vi "Basic_pn.vi"() -> ()   [LabVIEW 2019, in "GettingStarted_5775_Host.lvlib"]
uses:
  GettingStarted_5775_Host.lvlib
  <vilib>/userDefined/High Color/nirio_resource_hc.ctl
  <instrlib>/FlexRIO/API/Host/v1/NI FlexRIO/API/Reference Clock Source.ctl
  <instrlib>/FlexRIO/API/Host/v1/NI FlexRIO/API/Configure Reference Clock.vi
  <instrlib>/FlexRIO/API/Host/v1/NI FlexRIO/API/Get Property Reference - Fpga Small.vi
  <instrlib>/FlexRIO/API/Host/v1/NI FlexRIO/API/Configure Analog Start Trigger.vi
  <instrlib>/FlexRIO/API/Host/v1/NI FlexRIO/API/Configure Digital Edge Start Trigger.vi
  <instrlib>/FlexRIO/API/Host/v1/NI FlexRIO/API/Configure Immediate Start Trigger.vi
  <instrlib>/FlexRIO/API/Host/v1/NI FlexRIO/API/Read Stream 1D WDT.vi
  <vilib>/measure/maspectr.llb/FFT Power Spectrum and PSD for N Chan.vi
  <vilib>/FPGAPlugInAG/Dynamic/niLvFpga_Close_Dynamic.vi
  <vilib>/rvi/interface/nirviCloseFPGA/nirviCloseFPGA.xnode
  <instrlib>/FlexRIO/API/Host/v1/NI FlexRIO API v1.lvlib
  <resource>/objmgr/niflexrioapiStream.rc
  <vilib>/measure/NI_MAPro.lvlib
panel:
  in  "reference clock source":T1 items=["Default", "Onboard", "PXI_Clk10", "External", "None", "Baseboard Reference"]
  out "Sample Rate":dbl=3200000000.0 format="%#_6p"
  in  "ADC Interleaving Factor":i32=1 min=0 max=2 step=1
  in  "AI num samples":u64=320 step=16
  in  "AI channels":string="AI0,AI1"
  out "Device Power":dbl(slide) scale=-1.0..58.0 scale format="%#_3p"
  out "FPGA Temperature":dbl(slide) scale=0.0..100.0 scale format="%#_3p"
  in  "Trigger Type":enum32{"Immediate", "Analog", "Digital"}(tab)
  in  "trigger channel":string="AI0"
  in  "rising edge?":bool=TRUE
  in  "level (V)":dbl format="%#_3p"
  in  "hysteresis (V)":dbl format="%#_3p"
  in  "digital trigger source":string(combo)
  in  "stop":bool
  in  "Bitfile path":path
  in  "Waveform Tab Control":enum32{"AI Time Domain", "AI Frequency Domain"}(tab)
  out "Waveform Graph":waveform(dbl)[](graph)
  out "FFT":cluster{"f0":dbl, "df":dbl, "magnitude":dbl[]}[](graph) caption="Waveform Graph"
  out "error out":errorcluster
  out "Limit (W)":dbl
  out "Power (W)":dbl
  out "Limit (C)":dbl
  out "Temp (C)":dbl format="%#_4p"
  in  "RIO Device":T2
  # "Overview: Configure an acquisition for a FlexRIO target and transfer the data to the host using the FlexRIO Host API.  Loop an output waveform\nRequirements: FlexRIO\nInstructions: \n 1. Select the RIO Device that corresponds to the FlexRIO target. \n 2. Select the bitfile path that corresponds to your device\n 3. Optionally configure the clocking, stream, and trigger. \n 4. Run the VI"
  # "Resource Configuration"
  # "Clocking configuration"
  # "Input Waveform Configuration"
  # "Device Monitoring"
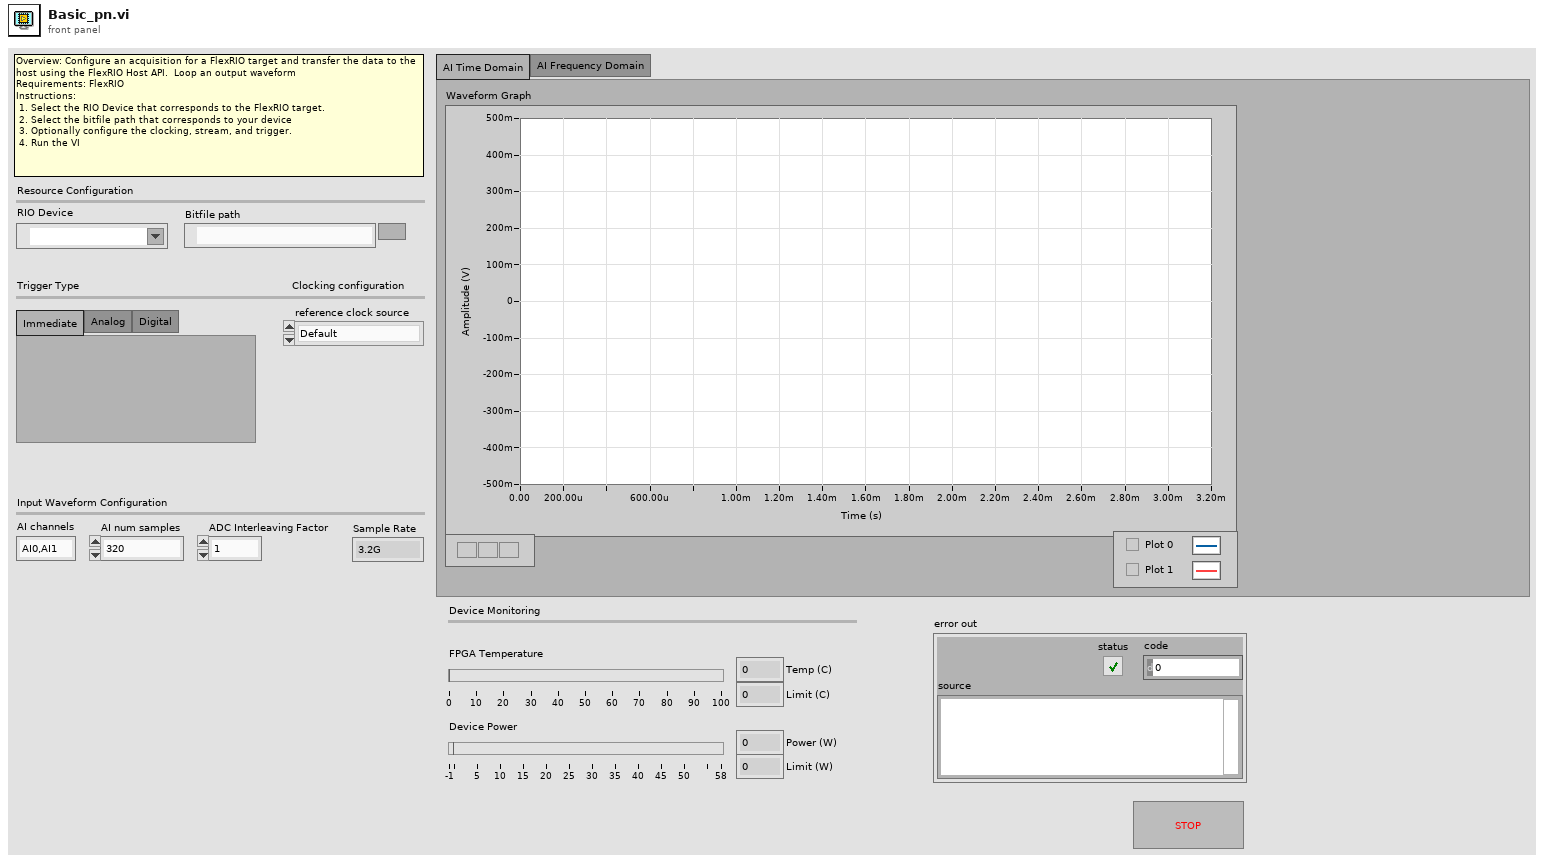
[diagram p1: front panel]
types:
  T1 = typedef "NI FlexRIO API v1.lvlib/Reference Clock Source.ctl" = i32
  T2 = typedef "nirio_resource_hc.ctl" = tag
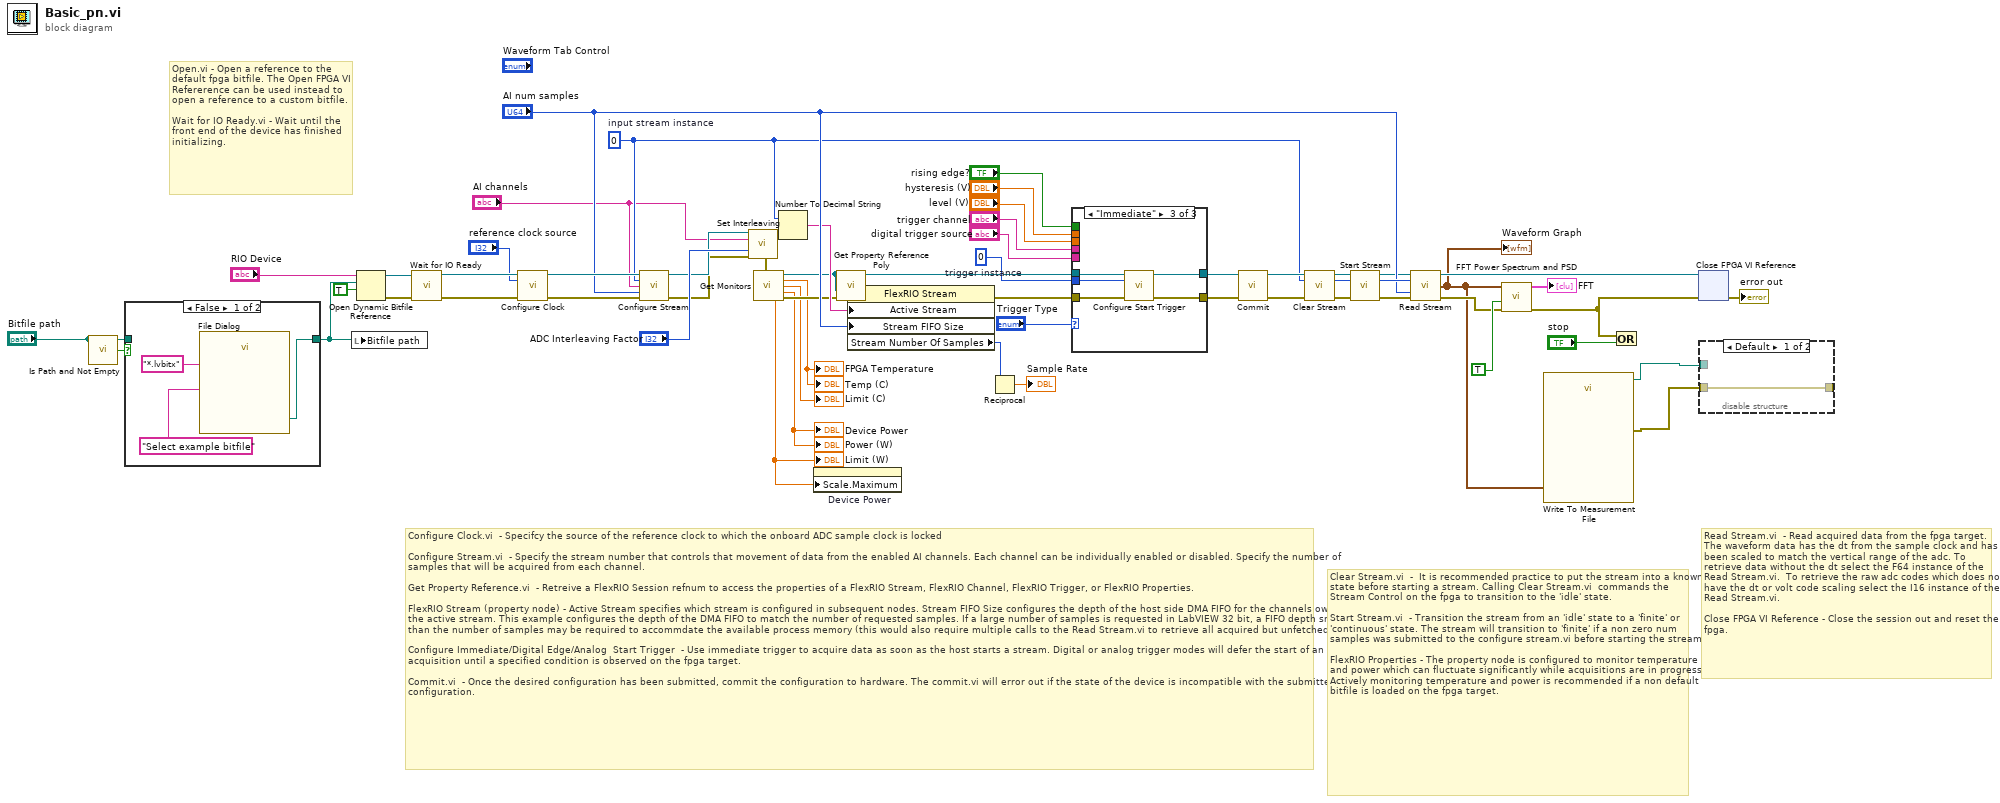
[diagram p0: block diagram]
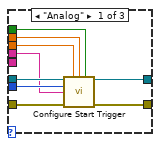
[diagram p2: hidden frame]
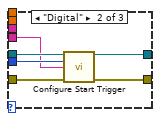
[diagram p3: hidden frame]
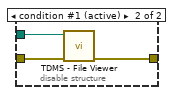
[diagram p4: hidden frame]
diagram:
  w32 = u32 0  # trigger instance
  w21 = u32 0  # input stream instance
  # "Read Stream.vi  - Read acquired data from the fpga target. The waveform data has the dt from the sample clock and has been scaled to match the vertical range of the adc. To retrieve data without the dt select the F64 instance of the Read Stream.vi.  To retrieve the raw adc codes which does not have the dt or volt code scaling select the I16 instance of the Read Stream.vi.  \n\nClose FPGA VI Reference - Close the session out and reset the fpga."
  # "Clear Stream.vi  -  It is recommended practice to put the stream into a known state before starting a stream. Calling Clear Stream.vi  commands the Stream Control on the fpga to transition to the 'idle' state.\n\nStart Stream.vi  - Transition the stream from an 'idle' state to a 'finite' or 'continuous' state. The stream will transition to 'finite' if a non zero num samples was submitted to the configure stream.vi before starting the stream.  \n\nFlexRIO Properties - The property node is configured to monitor temperature and power which can fluctuate significantly while acquisitions are in progress. Actively monitoring temperature and power is recommended if a non default bitfile is loaded on the fpga target."
  # "Configure Clock.vi  - Specifcy the source of the reference clock to which the onboard ADC sample clock is locked\n\nConfigure Stream.vi  - Specify the stream number that controls that movement of data from the enabled AI channels. Each channel can be individually enabled or disabled. Specify the number of samples that will be acquired from each channel. \n\nGet Property Reference.vi  - Retreive a FlexRIO Session refnum to access the properties of a FlexRIO Stream, FlexRIO Channel, FlexRIO Trigger, or FlexRIO Properties.\n\nFlexRIO Stream (property node) - Active Stream specifies which stream is configured in subsequent nodes. Stream FIFO Size configures the depth of the host side DMA FIFO for the channels owned by the active stream. This example configures the depth of the DMA FIFO to match the number of requested samples. If a large number of samples is requested in LabVIEW 32 bit, a FIFO depth smaller than the number of samples may be required to accommdate the available process memory (this would also require multiple calls to the Read Stream.vi to retrieve all acquired but unfetched data). \n\nConfigure Immediate/Digital Edge/Analog  Start Trigger  - Use immediate trigger to acquire data as soon as the host starts a stream. Digital or analog trigger modes will defer the start of an acquisition until a specified condition is observed on the fpga target. \n\nCommit.vi  - Once the desired configuration has been submitted, commit the configuration to hardware. The commit.vi will error out if the state of the device is incompatible with the submitted configuration."
  # "Open.vi - Open a reference to the default fpga bitfile. The Open FPGA VI Refererence can be used instead to open a reference to a custom bitfile.\n\nWait for IO Ready.vi - Wait until the front end of the device has finished initializing."
  n1 = call <vilib>:"Is Path and Not Empty.vi"("path"="Bitfile path") -> ("Is Path and Not Empty?"=w49:bool)  [unwired: 4 in]
  n2 = case shown="False" w49 {
    tunnel: "Bitfile path" -> [_ w63]
    tunnel: [w61 w63] -> w48
    frame False {
      n3 = call "File Dialog"("prompt"="Select example bitfile", "pattern (all files)"="*.lvbitx") -> ("selected path"=w61:path)  [unwired: 10 in, 3 out]
    }
    frame True {
    }
  }
  n4 = local write "Bitfile path"(w48) -> ()
  n5 = Open Dynamic Bitfile Reference(0:"RIO Device", 1:w48, 2:TRUE ("Run When Loaded")) -> (5:w55:refnum<k20>, 8:w56:errorcluster)  [unwired: 2 in]
  n6 = call <instrlib>:"Wait for IO Ready.vi"("fpga interface in"=w55, "error in"=w56) -> ("fpga interface out"=w57:refnum<k20>, "error out"=w58:errorcluster)  [unwired: 10 in, 2 out]
  n7 = call-poly <instrlib>:"Configure Clock.vi"("fpga interface in"=w57, "reference clock source"="reference clock source", "error in"=w58) -> ("fpga interface out"=w38:refnum<k20>, "error out"=w37:errorcluster)  [unwired: 11 in]
  n8 = call <instrlib>:"Configure Stream.vi"("fpga interface in"=w38, "stream instance"=w21, "channels enabled"="AI channels", "num samples"="AI num samples", "error in"=w37) -> ("fpga interface out"=w14:refnum<k20>, "error out"=w12:errorcluster)  [unwired: 7 in, 2 out]
  n9 = call "Set Interleaving.vi"("fpga interface in"=w14, "AI channels enabled"="AI channels", "ADC Interleaving Factor"="ADC Interleaving Factor", "error in (no error)"=w12) -> ("fpga interface out"=w15:refnum<k20>, "error out"=w16:errorcluster)  [unwired: 10 in]
  n10 = call "Get Monitors.vi"("fpga interface in"=w15, "error in (no error)"=w16) -> ("fpga interface out"=w8:refnum<k20>, "FPGA Temperature (C)"=→"Temp (C)" →"FPGA Temperature":dbl, "Temperature Limit (C)"=→"Limit (C)":dbl, "Total Power (W)"=→"Power (W)" →"Device Power":dbl, "Power Limit (W)"=w4:dbl, "error out"=w11:errorcluster)  [unwired: 8 in]
  "Limit (W)" <- w4
  n11 = Number To Decimal String(number=w21) -> (decimal integer string=w34:string)  [unwired: 1 in]
  n12 = property on="Device Power" class="Slide (strict)"("Scale.Maximum"=w4) -> ()  [unwired: 2 in, 2 out]
  n13 = call-poly <instrlib>:"Get Property Reference Poly.vi"("error in (no error)"=w11, "fpga interface in"=w8) -> ("error out"=w10:errorcluster, "property reference"=w9:refnum<k20>)  [unwired: 4 in, 1 out]
  n14 = property class="FlexRIO Stream"(reference=w9, error in=w10, "Active Stream"=w34, "Stream FIFO Size"="AI num samples") -> (error out=w27:errorcluster, "Stream Number Of Samples"=w20:u64)  [unwired: 1 out]
  n15 = Reciprocal(x=w20) -> (1/x=→"Sample Rate":dbl)
  n16 = case shown="\"Immediate\"" "Trigger Type" {
    tunnel: w8 -> [w72 w78 w83]
    tunnel: w27 -> [w71 w77 w82]
    tunnel: [w70 w76 w81] -> w26
    tunnel: [w69 w75 w80] -> w25
    tunnel: w32 -> [w68 w74 w79]
    tunnel: "trigger channel" -> [w67 _ _]
    tunnel: "level (V)" -> [w66 _ _]
    tunnel: "hysteresis (V)" -> [w65 _ _]
    tunnel: "rising edge?" -> [w64 _ _]
    tunnel: "digital trigger source" -> [_ w73 _]
    frame "Analog" {
      n17 = call-poly <instrlib>:"Configure Start Trigger.vi"("fpga interface in"=w72, "level"=w66, "hysteresis"=w65, "rising edge?"=w64, "trigger instance"=w68, "channel"=w67, "error in"=w71) -> ("fpga interface out"=w70:refnum<k20>, "error out"=w69:errorcluster)  [unwired: 6 in, 1 out]
    }
    frame "Digital" {
      n18 = call-poly <instrlib>:"Configure Start Trigger.vi"("fpga interface in"=w78, "trigger instance"=w74, "trigger source"=w73, "error in"=w77) -> ("fpga interface out"=w76:refnum<k20>, "error out"=w75:errorcluster)  [unwired: 9 in, 1 out]
    }
    frame "Immediate" {
      n19 = call-poly <instrlib>:"Configure Start Trigger.vi"("fpga interface in"=w83, "trigger instance"=w79, "error in"=w82) -> ("fpga interface out"=w81:refnum<k20>, "error out"=w80:errorcluster)  [unwired: 10 in, 1 out]
    }
  }
  n20 = call <instrlib>:"Commit.vi"("fpga interface in"=w26, "error in"=w25) -> ("fpga interface out"=w31:refnum<k20>, "error out"=w22:errorcluster)  [unwired: 12 in]
  n21 = call <instrlib>:"Clear Stream.vi"("fpga interface in"=w31, "stream instance"=w21, "error in"=w22) -> ("fpga interface out"=w41:refnum<k20>, "stream instance out"=w40:u32, "error out"=w39:errorcluster)  [unwired: 10 in]
  n22 = call <instrlib>:"Start Stream.vi"("fpga interface in"=w41, "stream instance"=w40, "error in"=w39) -> ("fpga interface out"=w24:refnum<k20>, "stream instance out"=w36:u32, "error out"=w23:errorcluster)  [unwired: 10 in]
  n23 = call-poly <instrlib>:"Read Stream.vi"("fpga interface in"=w24, "stream instance"=w36, "samples"="AI num samples", "error in"=w23) -> ("fpga interface out"=w52:refnum<k20>, "read data"=w1:waveform(dbl)[], "error out"=w18:errorcluster)  [unwired: 7 in, 2 out]
  "Waveform Graph" <- w1
  n24 = call-poly <vilib>:"FFT Power Spectrum and PSD.vi"("error in (no error)"=w18, "dB On (F)"=TRUE, "time signals"=w1) -> ("error out"=w51:errorcluster, "Power Spectrum / PSD"=→"FFT":cluster{"f0":dbl, "df":dbl, "magnitude":dbl[]}[])  [unwired: 5 in, 2 out]
  n25 = call "Write To Measurement File"("Signals"=w1) -> ("Filename Out"=w46:path, "error out"=w47:errorcluster)  [unwired: 16 in, 1 out]
  n26 = Or(x=w51, y="stop") -> ()  [unwired: 1 out]
  n27 = xnode "Close FPGA VI Reference"("FPGA VI Reference In"=w52, "error in"=w51) -> ("error out"=→"error out":errorcluster)
  n28 = disable-structure shown="Default" {
    disable-tunnel: w46 -> [_ w87]
    disable-tunnel: [w84 w86] -> _
    disable-tunnel: w47 -> [w84 w85]
    frame condition #0 {
    }
    frame condition #1 (active) {
      n29 = call <vilib>:"TDMS - File Viewer.vi"("error in (no error)"=w85, "file path"=w87) -> ("error out"=w86:errorcluster)  [unwired: 5 out]
    }
  }
